vi "Sub_Electrical_Noise_Analysis-Excel-1.vi"(10 "Init Col Value":i32, 11 "Init Row Value":i32) -> (3 "Output":string[][](array[string]))   [LabVIEW 2015]
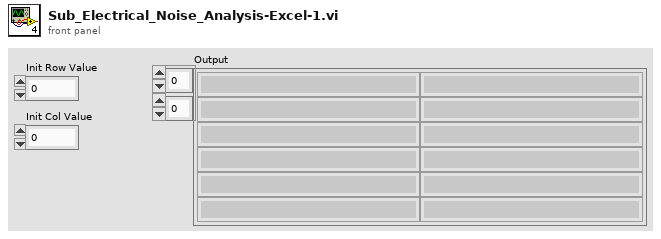
[diagram p1: front panel]
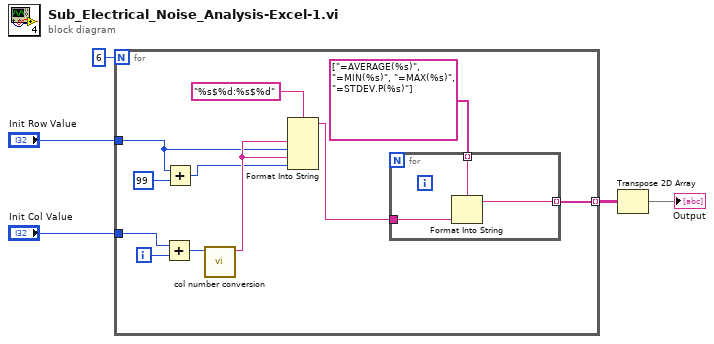
[diagram p0: block diagram]
diagram:
  n1 = for {
    N: 6 -> [_]
    tunnel: "Init Col Value" -> [w14]
    tunnel: "Init Row Value" -> [w9]
    tunnel: [w6] -> w2 mode=indexing
    i -> [w15]
    n2 = Add(x=w14, y=w15) -> (x+y=w11:i32)
    n3 = Add(x=w9, y=99) -> (x+y=w8:i32)
    n4 = call "col number conversion.vi"("Col Number"=w11) -> ("Excel Col Number"=w10:string)  [unwired: 10 in]
    n5 = Format Into String(format string="%s$%d:%s$%d" ("포맷 문자열"), w10, w9, w10, w8) -> (resulting string=w7:string)  [unwired: 2 in, 1 out]
    n6 = for {
      tunnel: string[] ["=AVERAGE(%s)", "=MIN(%s)", "=MAX(%s)", "=STDEV.P(%s)"] -> [w19] mode=indexing
      tunnel: w7 -> [w18]
      tunnel: [w17] -> w6 mode=indexing
      n7 = Format Into String(format string=w19, w18) -> (resulting string=w17:string)  [unwired: 2 in, 1 out]
    }
  }
  n8 = Transpose 2D Array(2D array=w2) -> (transposed array=→"Output":string[][])
